vi "HMI.vi"() -> ()   [LabVIEW 2022 SP3]
uses:
  <vilib>/Instr/_visa.llb/VISA Configure Serial Port (Instr).vi
panel:
  out "Longitud":dbl
  out "Latitud":dbl
  out "Time Stamp":timestamp
  out "Altura Aprox en m":dbl(slide) scale=0.0..14000.0
  out "Presion en Pa":dbl(knob) scale=0.0..100000.0
  out "Temperatura en C":dbl(slide) scale=-30.0..100.0
  in  "stop":bool
  out "Datos recibidos":string
  in  "VISA resource name":refnum<visa-resource-name>
  # "PROYECTO FINAL ADQUISION DE DATOS"
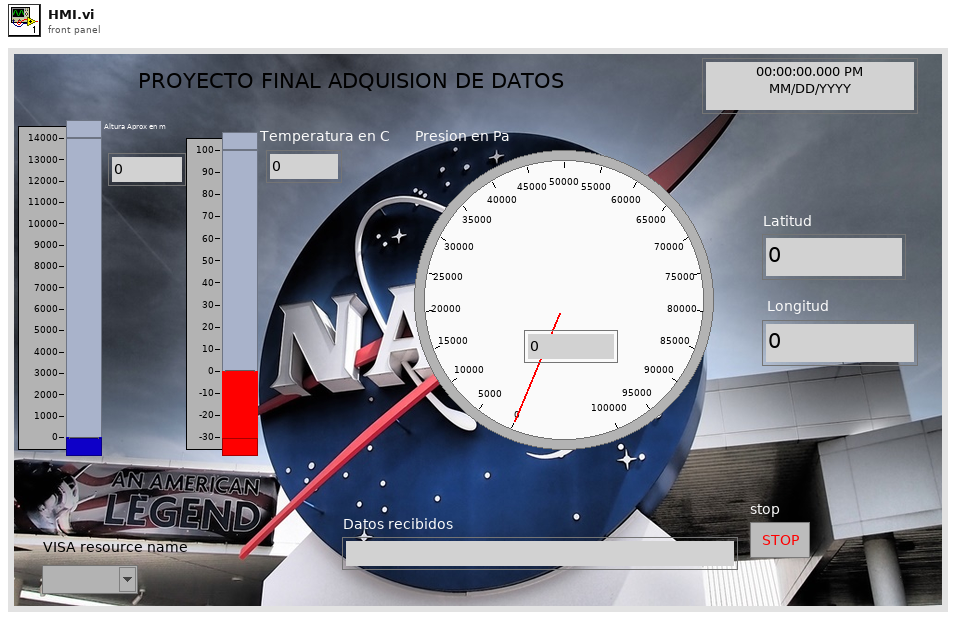
[diagram p1: front panel]
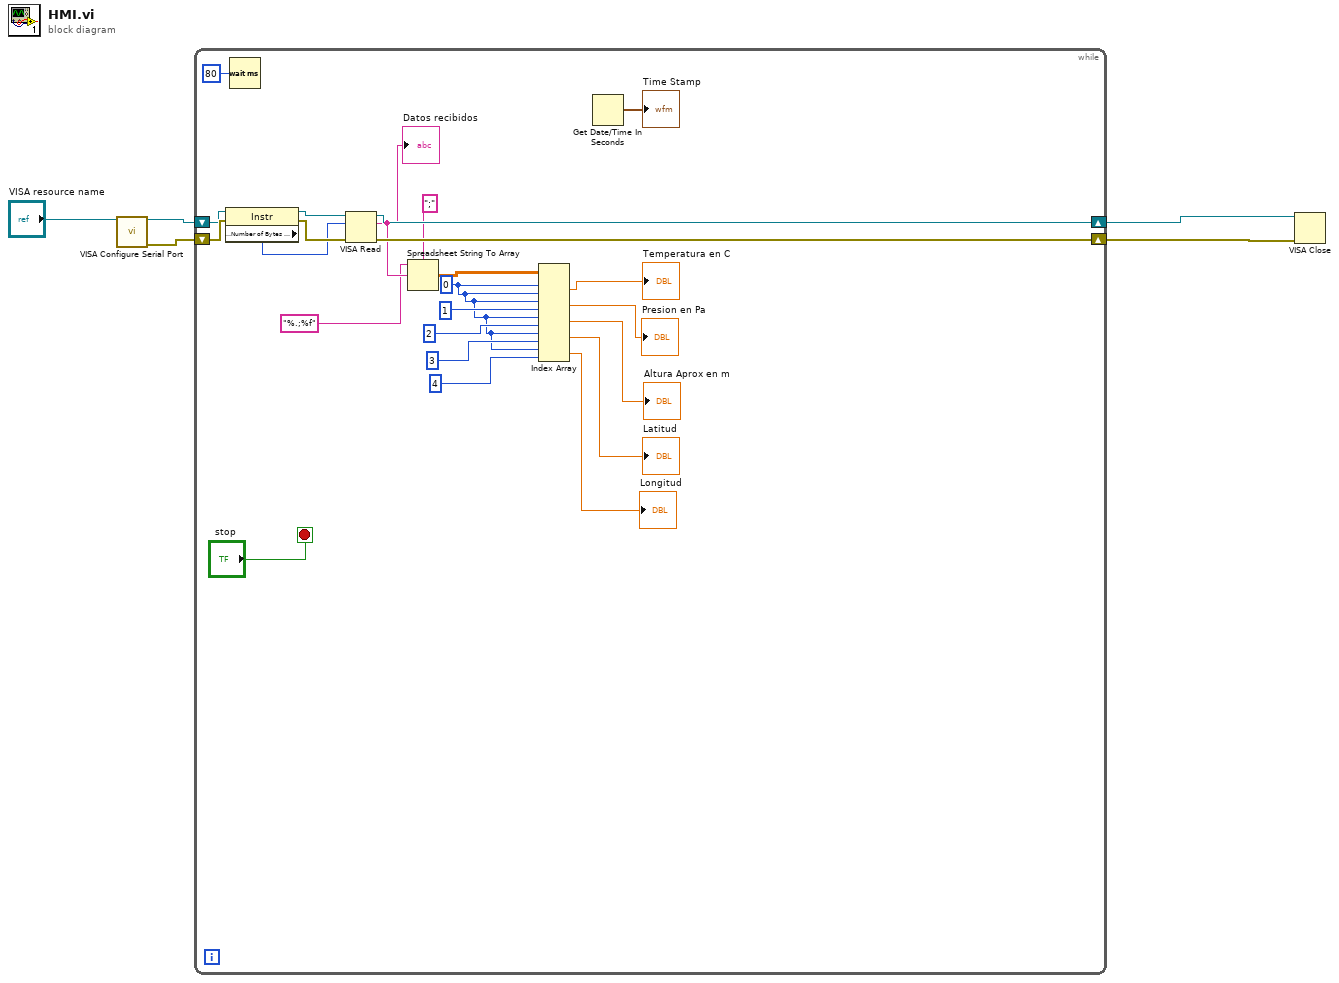
[diagram p0: block diagram]
diagram:
  n1 = call-poly "VISA Configure Serial Port"("VISA resource name"="VISA resource name") -> ("VISA resource name out"=w4:refnum<visa-resource-name>, "error out"=w5:errorcluster)  [unwired: 13 in]
  n2 = while {
    shift-right: [w23] -> w1
    shift-left: w5 -> [w26]
    shift-right: [w24] -> w2
    shift-left: w4 -> [w25]
    stop <- "stop" stop-if-true
    w12 = 0 ("index (row)")
    n3 = property class="Instr"(reference=w25, error in=w26) -> (reference out=w29:refnum<visa-resource-name>, error out=w28:errorcluster, "Serial Settings:Number of Bytes at Serial Port"=w27:u32)
    n4 = Wait (ms)(milliseconds to wait=u32 80) -> ()  [unwired: 1 out]
    n5 = VISA Read(VISA resource name=w29, byte count=w27, error in (no error)=w28) -> (VISA resource name out=w24:refnum<visa-resource-name>, read buffer=w20:string, error out=w23:errorcluster)  [unwired: 1 out]
    "Datos recibidos" <- w20
    n6 = Spreadsheet String To Array(delimiter (Tab)=";", format string="%.;%f", spreadsheet string=w20) -> (array=w17:dbl[][])  [unwired: 1 in]
    n7 = Index Array(array=w17, index (row) #1=w12, index (col) #1=w12, index (row) #2=w12, index (col) #2=1 ("disabled index (col)"), index (row) #3=w12, index (col) #3=2 ("index (row)"), index (row) #4=w12, index (col) #4=3 ("disabled index (col)"), index (row) #5=w12, index (col) #5=4 ("disabled index (col)")) -> (element #1=→"Temperatura en C":dbl, element #2=→"Presion en Pa":dbl, element #3=→"Altura Aprox en m":dbl, element #4=→"Latitud":dbl, element #5=→"Longitud":dbl)
    n8 = Get Date/Time In Seconds() -> (seconds since 1Jan1904=→"Time Stamp":timestamp)
  }
  n9 = VISA Close(VISA resource name=w2, error in (no error)=w1) -> ()  [unwired: 1 out]
